vi "encodeInt16.vi"(2 "Compress? (T)":bool=TRUE, 3 "Int16":i16) -> (1 "MessagePack":u8[](array[numeric]) format="%.0x")   [LabVIEW 2015, in "MsgPack.lvlib"]
uses:
  MsgPack.lvlib
  SubVis/encodeFixedInt.vi
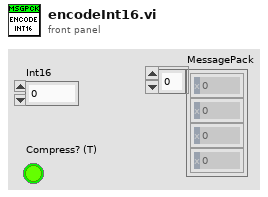
[diagram p1: front panel]
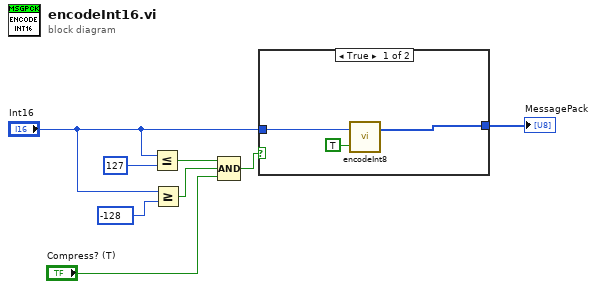
[diagram p0: block diagram]
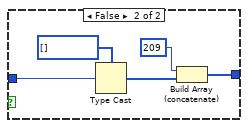
[diagram p2: hidden frame]
diagram:
  n1 = Less Or Equal?(x="Int16", y=i16 127) -> (x <= y?=w5:bool)
  n2 = Greater Or Equal?(x="Int16", y=i16 -128) -> (x >= y?=w4:bool)
  n3 = Compound Arithmetic op=AND(w5, w4, "Compress? (T)") -> (w2:bool)
  n4 = case shown="True" w2 {
    tunnel: [w11 w16] -> w8
    tunnel: "Int16" -> [w10 w12]
    frame True {
      n5 = call "encodeInt8.vi"("Compress? (T)"=TRUE ("Compress"), "Int8"=w10) -> ("MessagePack"=w11:u8[])  [unwired: 1 in]
    }
    frame False {
      n6 = Type Cast(type=u8[] [], x=w12) -> (*(type *) &x=w13:u8[])
      n7 = Build Array (concatenate)(u8 209, w13) -> (w16:u8[])
    }
  }
  "MessagePack" <- w8
